vi "PCU_Get_LAN_Portnumber.vi"(8 "error in (no error)":errorcluster, 11 ".NET Reference in":refnum<k24>) -> (0 "error out":errorcluster, 2 "port":i32, 3 "Reference out":refnum<k24>)   [LabVIEW 2017]
uses:
  C:/Users/Ssantec_Test/Documents/Instrument_DLL_Sample_Labview_20220902_Ver1.2.2/DLL/x86/InstrumentDLL.dll
  DLL/x86/InstrumentDLL.dll
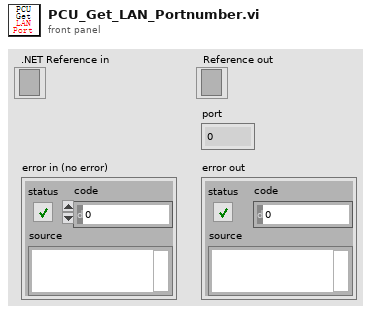
[diagram p1: front panel]
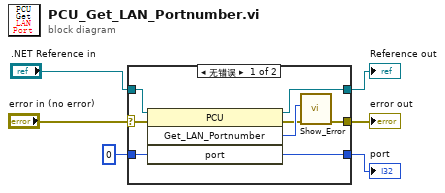
[diagram p0: block diagram]
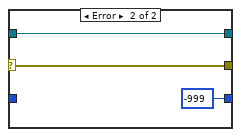
[diagram p2: hidden frame]
diagram:
  n1 = case shown="无错误" "error in (no error)" {
    selector: "error in (no error)" -> [w7 w16]
    tunnel: [w14 -999 ("port")] -> w6
    tunnel: 0 ("port") -> [w13 _]
    tunnel: ".NET Reference in" -> [w12 w17]
    tunnel: [w8 w16] -> w3
    tunnel: [w11 w17] -> w2
    frame No Error {
      n2 = invoke on="调用节点" class="PCU" method="Get_LAN_Portnumber"(reference=w12, error in=w7, "port"=w13) -> (reference out=w11:refnum<k24>, error out=w9:errorcluster, "Get_LAN_Portnumber"=w10:i32, "port"=w14:i32)  [unwired: 1 in]
      n3 = call "Show_Error.vi"("error in (no error)"=w9, "Error"=w10) -> ("error out"=w8:errorcluster)  [unwired: 9 in]
    }
    frame Error {
    }
  }
  "port" <- w6
  "error out" <- w3
  "Reference out" <- w2
